vi "FindMatlabBoundControlByName.vi"(10 "name":string, 11 "ExperimentID":string) -> (1 "AllowVariantValues":bool, 2 "Boolean":bool, 3 "Control out":refnum<vi>)   [LabVIEW 2017]
uses:
  Types/MatlabBindingDirectionEnum.ctl
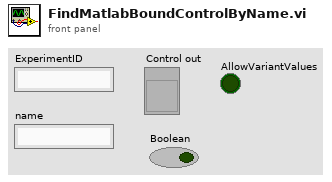
[diagram p1: front panel]
types:
  T1 = typedef "ControlValueChangeEventBindingType.ctl" = cluster{"Control":refnum<vi>, "Event Register":refnum<event-registration>, "AllowVariantValues":bool, "Direction":T2}
  T2 = typedef "MatlabBindingDirectionEnum.ctl" = enum16{"BiDirectional", "FromMatlab", "ToMatlab"}
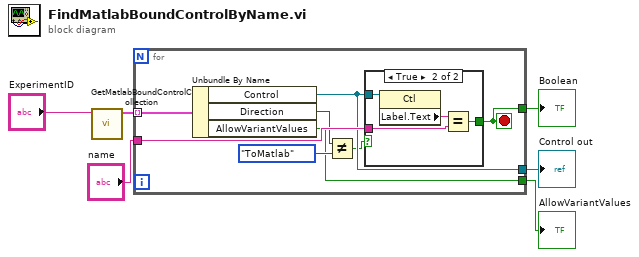
[diagram p0: block diagram]
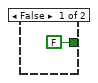
[diagram p2: hidden frame]
diagram:
  n1 = call "GetMatlabBoundControlCollection.vi"("ExpID"="ExperimentID") -> ("Bound Controls"=w3:T1[])  [unwired: 10 in]
  n2 = for {
    tunnel: w3 -> [w14] mode=indexing
    tunnel: "name" -> [w13]
    tunnel: [w12] -> w5
    tunnel: [w11] -> w6
    tunnel: [w7] -> w1
    stop <- w11 stop-if-true
    n3 = Unbundle By Name(w14) -> ("Control"=w12:refnum<vi>, "Direction"=w10:T2, "AllowVariantValues"=w7:bool)
    n4 = Not Equal?(x=w10, y=MatlabBindingDirectionEnum."ToMatlab") -> (x != y?=w8:bool)
    n5 = case shown="True" w8 {
      tunnel: w13 -> [_ w18]
      tunnel: w12 -> [_ w17]
      tunnel: [FALSE w16] -> w11
      frame False {
      }
      frame True {
        n6 = property class="Ctl"(reference=w17) -> ("Label.Text"=w19:string)  [unwired: 1 in, 2 out]
        n7 = Equal?(x=w19, y=w18) -> (x = y?=w16:bool)
      }
    }
  }
  "Boolean" <- w6
  "Control out" <- w5
  "AllowVariantValues" <- w1
